vi "Term_Project.vi"() -> ()   [LabVIEW 2014]
doc: "This VI illustrates how to perform simultaneous sound IO, i.e., how to continuously play the sound acquired from a microphone. It requires the use of a microphone attached to the sound card. You can specify the IDs of the input and output devices, the frequency to sample at, and the buffer size for both devices. Higher frequencies have better quality, but demand more resources and are limited by the capabilities of your sound card. A large number of samples decreases the risk of glitches, but increases the delay between acquisition and playback."
uses:
  <vilib>/sound2/lvsound2.llb/Sampling Mode.ctl
  <vilib>/sound2/lvsound2.llb/Sound Data Format.ctl
  <vilib>/Analysis/3filter.llb/Filter Passband Type.ctl
  <vilib>/Analysis/baseanly.llb/Quick Scale 1D.vi
  <vilib>/sound2/lvsound2.llb/Sound Output Write (DBL Single).vi
  <instrlib>/niUSRP/niUSRP Fetch Rx Data (CDB WDT).vi
  <vilib>/Analysis/3filter.llb/Butterworth Filter (DBL).vi
  <vilib>/sound2/lvsound2.llb/Sound Input Read (DBL).vi
  <vilib>/imath/engines/lvmath2/RunTimeEngine/BuiltInFunctions/abs/NIMS_abs(signed).vi
  <instcachedir>/0/NIMS_abs(signed)_C4FCB8E6058B49B797C7C8D53CA5F6EC.lvgen/NIMS_abs(signed)_C4FCB8E6058B49B797C7C8D53CA5F6EC_001.vi
  <vilib>/imath/engines/lvmath2/RunTimeEngine/BuiltInFunctions/max/1 input/NIMS_max(RV).vi
  <instcachedir>/0/NIMS_max(RV)_237633DB1D604D5BA7001287DF3C7957.lvgen/NIMS_max(RV)_237633DB1D604D5BA7001287DF3C7957_000.vi
  <vilib>/imath/engines/lvmath2/RunTimeEngine/NodeEndStatement/NIMS_NodeEndStatement_Output.vi
  <instcachedir>/0/NIMS_NodeEndStatement_Output_53EC0D466D134D7ABD903AC30B43404B.lvgen/NIMS_NodeEndStatement_Output_53EC0D466D134D7ABD903AC30B43404B_000.vi
  <instcachedir>/0/NIMS_NodeEndStatement_Output_53EC0D466D134D7ABD903AC30B43404B.lvgen/NIMS_NodeEndStatement_Output_53EC0D466D134D7ABD903AC30B43404B_005.vi
  <vilib>/imath/engines/lvmath2/RunTimeEngine/ErrorHandling/NIMS_Finalize Error.vi
  <instrlib>/niUSRP/niUSRP Write Tx Data (CDB).vi
  <vilib>/Analysis/NI_AALBase.lvlib
panel:
  in  "active antenna (Rx)":string="RX2"
  out "actual gain (dB) (Rx)":dbl format="%#_6f"
  in  "gain (dB) (Rx)":dbl format="%#_6f"
  out "actual carrier frequency (Rx)":dbl=100000.0 format="%#_6p"
  out "actual IQ rate (Rx)":dbl=100000.0 format="%#_6p"
  in  "IQ rate (Rx)":dbl=1000000.0 format="%#_6p"
  in  "Rx device":refnum<k15>="192.168.10.2"
  in  "carrier frequency":u16(ring) items=["151.6550 MHz", "151.6850 MHz", "151.7150 MHz"]
  out "Baseband Output":dbl[](graph)
  in  "active antenna (Tx)":string="TX1"
  out "actual gain (dB) (Tx)":dbl format="%#_6f"
  in  "gain (dB) (Tx)":dbl format="%#_6f"
  out "actual carrier frequency (Tx)":dbl=100000.0 format="%#_6p"
  out "actual IQ rate (Tx)":dbl=100000.0 format="%#_6p"
  in  "IQ rate (Tx)":dbl=200000.0 format="%#_6p"
  in  "Tx device":refnum<k15>="192.168.10.2"
  out "Baseband Signal":dbl[](graph)
  out "Message":waveform(dbl)[](graph)
  in  "Modulation index":dbl(slide)=1.0 min=0.0 max=1.0 scale=0.0..1.0
  in  "Record":bool
  in  "Stop":bool
  in  "Input Device ID":u32
  in  "Output Device ID":u32
  # "TRANSMITTING"
  # "CONTROL"
  # "RECEIVING"
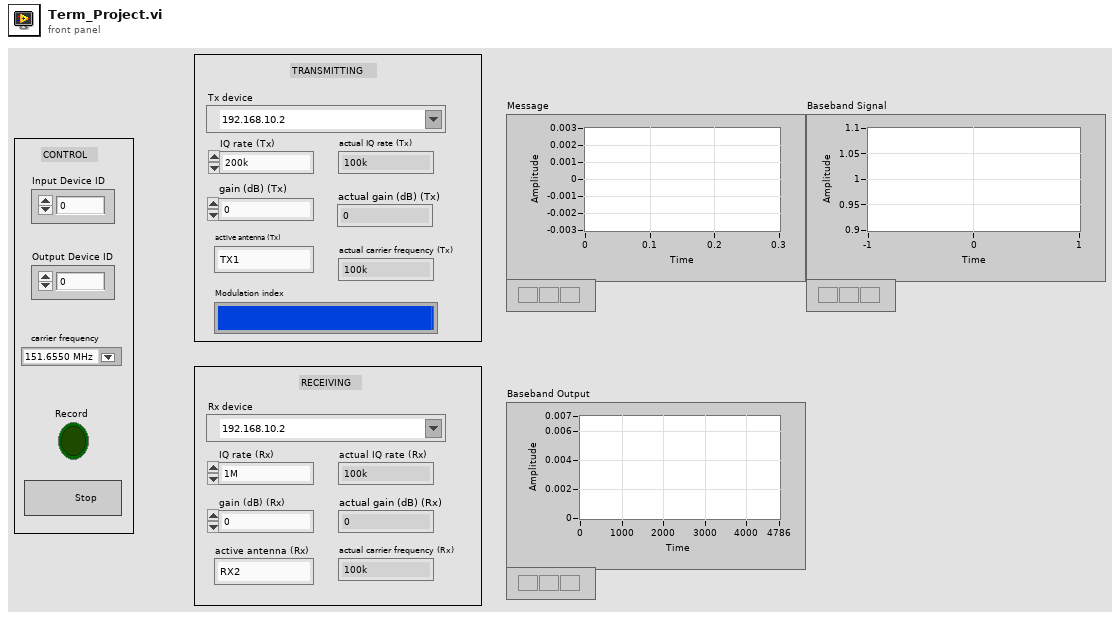
[diagram p1: front panel]
types:
  T1 = typedef "Sound Data Format.ctl" = cluster{"sample rate (S/s)":dbl, "number of channels":i32, "bits per sample":i32}
  T2 = typedef "Sampling Mode.ctl" = i32
  T3 = typedef "Sound Output Task ID.ctl" = u32
  T4 = typedef "Sound Input Task ID.ctl" = u32
  T5 = typedef "NI_AALBase.lvlib/Filter Passband Type.ctl" = enum32{"Lowpass", "Highpass", "Bandpass", "Bandstop"}
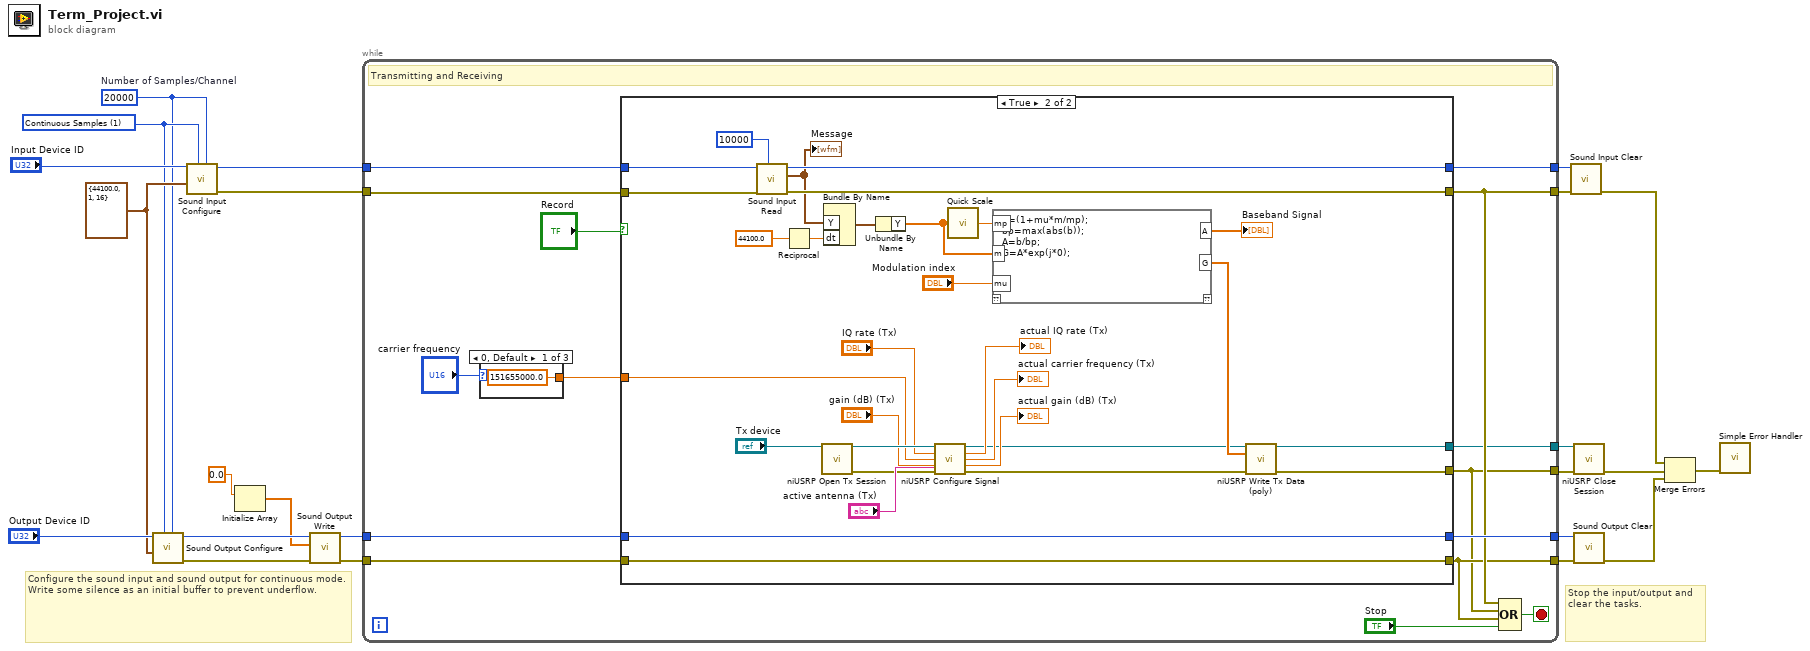
[diagram p0: block diagram]
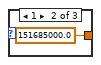
[diagram p2: hidden frame]
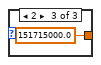
[diagram p3: hidden frame]
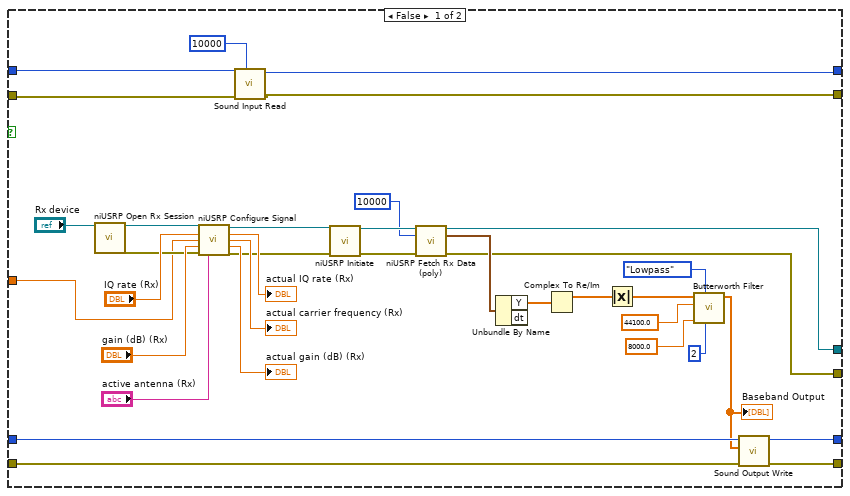
[diagram p4: hidden frame]
diagram:
  w4 = 20000  # Number of Samples/Channel
  w9 = T1 {"sample rate (S/s)"=44100.0, "number of channels"=1, "bits per sample"=16} ("Sound Format")
  w5 = T2 1 items=["Finite Samples", "Continuous Samples"] ("sample mode")
  # "Stop the input/output and clear the tasks."
  # "Configure the sound input and sound output for continuous mode. Write some silence as an initial buffer to prevent underflow."
  n1 = call <vilib>:"Sound Output Configure.vi"("number of samples/ch"=w4, "sample mode"=w5, "sound format"=w9, "device ID"="Output Device ID") -> ("error out"=w13:errorcluster, "task ID"=w14:T3)  [unwired: 6 in]
  n2 = call <vilib>:"Sound Input Configure.vi"("number of samples/ch"=w4, "sample mode"=w5, "sound format"=w9, "device ID"="Input Device ID") -> ("error out"=w16:errorcluster, "task ID"=w15:T4)  [unwired: 6 in]
  n3 = Initialize Array(0.0 ("element")) -> (w7:dbl[])  [unwired: 1 in]
  n4 = call-poly <vilib>:"Sound Output Write.vi"("error in (no error)"=w13, "data"=w7, "task ID"=w14) -> ("error out"=w12:errorcluster, "task ID out"=w11:T3)  [unwired: 7 in]
  n5 = while {
    tunnel: w15 -> [w31]
    tunnel: [w36] -> w18
    tunnel: w11 -> [w38]
    tunnel: [w37] -> w21
    tunnel: w12 -> [w35]
    tunnel: [w25] -> w22
    tunnel: w16 -> [w30]
    tunnel: [w33] -> w23
    tunnel: [w24] -> w3
    tunnel: [w26] -> w1
    stop <- w34 stop-if-true
    # "Transmitting and Receiving"
    n6 = case shown="0, Default" "carrier frequency" {
      tunnel: [151655000.0 ("sample rate (S/s)") 151685000.0 ("sample rate (S/s)") 151715000.0 ("sample rate (S/s)")] -> w27
      frame 0, Default {
      }
      frame 1 {
      }
      frame 2 {
      }
    }
    n7 = case shown="True" "Record" {
      tunnel: w38 -> [w69 w78]
      tunnel: [w71 w78] -> w37
      tunnel: [w76 w106] -> w36
      tunnel: w35 -> [w68 w77]
      tunnel: [w70 w77] -> w25
      tunnel: [w75 w105] -> w33
      tunnel: w30 -> [w73 w103]
      tunnel: w31 -> [w74 w102]
      tunnel: [w43 w79] -> w26
      tunnel: [w42 w80] -> w24
      tunnel: w27 -> [w44 w81]
      frame False {
        n8 = call <instrlib>:"niUSRP Open Rx Session.vi"("device names"="Rx device") -> ("session handle out"=w45:refnum<k15>, "error out"=w46:errorcluster)  [unwired: 13 in]
        n9 = call <instrlib>:"niUSRP Configure Signal.vi"("session handle"=w45, "IQ rate"="IQ rate (Rx)", "carrier frequency"=w44, "gain"="gain (dB) (Rx)", "error in (no error)"=w46, "active antenna"="active antenna (Rx)") -> ("session handle out"=w48:refnum<k15>, "coerced IQ rate"=→"actual IQ rate (Rx)":dbl, "coerced carrier frequency"=→"actual carrier frequency (Rx)":dbl, "coerced gain"=→"actual gain (dB) (Rx)":dbl, "error out"=w47:errorcluster)  [unwired: 5 in]
        n10 = call-poly <vilib>:"Sound Input Read.vi"("number of samples/ch"=10000, "error in (no error)"=w73, "task ID"=w74) -> ("error out"=w75:errorcluster, "task ID out"=w76:T4)  [unwired: 6 in, 1 out]
        n11 = call <instrlib>:"niUSRP Initiate.vi"("session handle"=w48, "error in (no error)"=w47) -> ("session handle out"=w67:refnum<k15>, "error out"=w66:errorcluster)  [unwired: 12 in]
        n12 = call-poly <instrlib>:"niUSRP Fetch Rx Data (poly).vi"("session handle"=w67, "number of samples"=i64 10000, "error in (no error)"=w66) -> ("session handle out"=w43:refnum<k15>, "data"=w64:waveform(cdb), "error out"=w42:errorcluster)  [unwired: 9 in, 1 out]
        n13 = Unbundle By Name(w64) -> ("Y"=w63:cdb[])  [unwired: 1 out]
        n14 = Complex To Re/Im(x + iy=w63) -> (x=w62:dbl[])  [unwired: 1 out]
        n15 = Absolute Value(x=w62) -> (abs(x)=w61:dbl[])
        n16 = call-poly <vilib>:"Butterworth Filter.vi"("order"=2, "filter type"=Filter_Passband_Type."Lowpass", "low cutoff freq: fl"=8000.0, "sampling freq: fs"=44100.0, "X"=w61) -> ("Filtered X"=w56:dbl[])  [unwired: 3 in, 1 out]
        "Baseband Output" <- w56
        n17 = call-poly <vilib>:"Sound Output Write.vi"("error in (no error)"=w68, "data"=w56, "task ID"=w69) -> ("error out"=w70:errorcluster, "task ID out"=w71:T3)  [unwired: 7 in]
      }
      frame True {
        n18 = call-poly <vilib>:"Sound Input Read.vi"("number of samples/ch"=10000, "error in (no error)"=w103, "task ID"=w102) -> ("error out"=w105:errorcluster, "data"=w96:waveform(dbl)[], "task ID out"=w106:T4)  [unwired: 6 in]
        "Message" <- w96
        n19 = Reciprocal(x=44100.0) -> (1/x=w94:dbl)
        n20 = call <instrlib>:"niUSRP Open Tx Session.vi"("device names"="Tx device") -> ("session handle out"=w92:refnum<k15>, "error out"=w88:errorcluster)  [unwired: 13 in]
        n21 = Bundle By Name("Y"=w96, "dt"=w94) -> (w97:waveform(dbl))  [unwired: 1 in]
        n22 = Unbundle By Name(w97) -> ("Y"=w98:dbl[])
        n23 = call <instrlib>:"niUSRP Configure Signal.vi"("session handle"=w92, "IQ rate"="IQ rate (Tx)", "carrier frequency"=w81, "gain"="gain (dB) (Tx)", "error in (no error)"=w88, "active antenna"="active antenna (Tx)") -> ("session handle out"=w83:refnum<k15>, "coerced IQ rate"=→"actual IQ rate (Tx)":dbl, "coerced carrier frequency"=→"actual carrier frequency (Tx)":dbl, "coerced gain"=→"actual gain (dB) (Tx)":dbl, "error out"=w82:errorcluster)  [unwired: 5 in]
        n24 = call-poly <vilib>:"Quick Scale.vi"("X"=w98) -> ("max|X|"=w100:dbl)  [unwired: 2 out]
        n25 = mathscript code="b=(1+mu*m/mp);\nbp=max(abs(b));\nA=b/bp;\nG=A*exp(j*0);"("mp"=w100, "m"=w98, "mu"="Modulation index") -> ("A"=→"Baseband Signal":dbl[], "G"=w95:cdb[])  [unwired: 1 in, 1 out]
        n26 = call-poly <instrlib>:"niUSRP Write Tx Data (poly).vi"("session handle"=w83, "data"=w95, "error in (no error)"=w82) -> ("session handle out"=w79:refnum<k15>, "error out"=w80:errorcluster)  [unwired: 11 in]
      }
    }
    n27 = Compound Arithmetic op=OR(w33, w24, w25, "Stop") -> (w34:bool)
  }
  n28 = call <vilib>:"Sound Input Clear.vi"("error in (no error)"=w23, "task ID"=w18) -> ("error out"=w17:errorcluster)  [unwired: 9 in]
  n29 = call <instrlib>:"niUSRP Close Session.vi"("session handle"=w1, "error in (no error)"=w3) -> ("error out"=w2:errorcluster)  [unwired: 13 in]
  n30 = call <vilib>:"Sound Output Clear.vi"("error in (no error)"=w22, "task ID"=w21) -> ("error out"=w6:errorcluster)  [unwired: 9 in]
  n31 = Merge Errors(w17, w2, w6) -> (w10:errorcluster)
  n32 = call <vilib>:"Simple Error Handler.vi"("error in (no error)"=w10) -> ()  [unwired: 4 in, 5 out]
